vi "Motion_Pulse Coils.vi"(8 "error in":errorcluster, 10 "Pulse Coil":T1=1 items=["GANTRY_ALARM_CLEAR", "GANTRY_ENABLE", "GANTRY_HOME", "GANTRY_GOTO", "LOADER_HOME", "LOADER_ALARM_CLEAR", "LOADER_ENABLE", "LOADER_GOTO_CONNECT", "LOADER_GOTO_LOAD", "LOADER_STOP"], 11 "TCP refnum":refnum<k5>) -> (0 "error out":errorcluster, 3 "TCP refnum dup":refnum<k5>)   [LabVIEW 2010]
uses:
  Motion_Coils Typedef.ctl
  <vilib>/NI Modbus.llb/MB Ethernet Master Query Write Single Coil (poly).vi
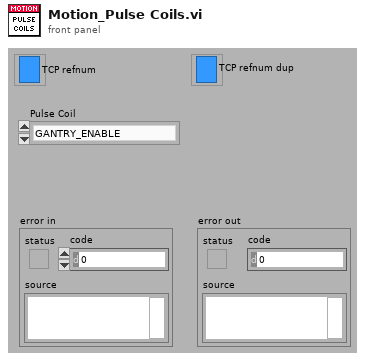
[diagram p1: front panel]
types:
  T1 = typedef "Motion_Coils Typedef.ctl" = u16
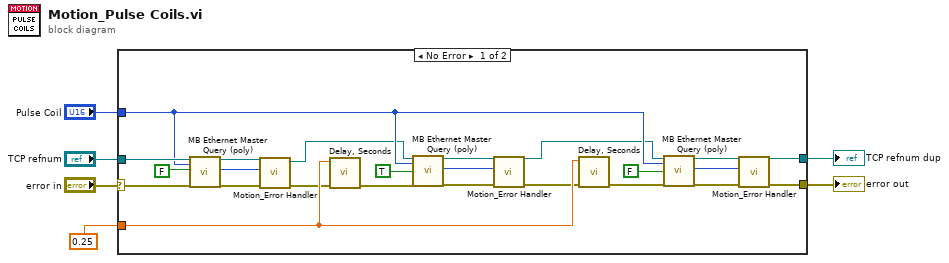
[diagram p0: block diagram]
diagram:
  n1 = case shown="No Error" "error in" {
    selector: "error in" -> [w23 w32]
    tunnel: "Pulse Coil" -> [w22 _]
    tunnel: dbl[unit] 0.25 ("delay") -> [w26 _]
    tunnel: [w13 w32] -> w5
    tunnel: "TCP refnum" -> [w25 w31]
    tunnel: [w11 w31] -> w1
    frame No Error {
      n2 = call-poly <vilib>:"MB Ethernet Master Query (poly).vi"("TCP Connection Refnum in"=w25, "Address"=w22, "Coil"=FALSE, "error in"=w23) -> ("TCP Connection Refnum (dup)"=w21:refnum<k5>, "Exception Code"=w19:u8, "error out"=w18:errorcluster)  [unwired: 13 in]
      n3 = call "Motion_Error Handler.vi"("error in (no error)"=w18, "Exception Code"=w19, "TCP Connection Refnum in"=w21) -> ("error out"=w17:errorcluster, "TCP Connection Refnum (dup)"=w20:refnum<k5>)  [unwired: 7 in]
      n4 = call "Delay, Seconds.vi"("error in"=w17, "delay"=w26) -> ("error out"=w27:errorcluster)  [unwired: 5 in, 1 out]
      n5 = call-poly <vilib>:"MB Ethernet Master Query (poly).vi"("TCP Connection Refnum in"=w20, "Address"=w22, "Coil"=TRUE, "error in"=w27) -> ("TCP Connection Refnum (dup)"=w8:refnum<k5>, "Exception Code"=w9:u8, "error out"=w16:errorcluster)  [unwired: 13 in]
      n6 = call "Motion_Error Handler.vi"("error in (no error)"=w16, "Exception Code"=w9, "TCP Connection Refnum in"=w8) -> ("error out"=w15:errorcluster, "TCP Connection Refnum (dup)"=w7:refnum<k5>)  [unwired: 7 in]
      n7 = call "Delay, Seconds.vi"("error in"=w15, "delay"=w26) -> ("error out"=w29:errorcluster)  [unwired: 5 in, 1 out]
      n8 = call-poly <vilib>:"MB Ethernet Master Query (poly).vi"("TCP Connection Refnum in"=w7, "Address"=w22, "Coil"=FALSE, "error in"=w29) -> ("TCP Connection Refnum (dup)"=w12:refnum<k5>, "Exception Code"=w10:u8, "error out"=w14:errorcluster)  [unwired: 13 in]
      n9 = call "Motion_Error Handler.vi"("error in (no error)"=w14, "Exception Code"=w10, "TCP Connection Refnum in"=w12) -> ("error out"=w13:errorcluster, "TCP Connection Refnum (dup)"=w11:refnum<k5>)  [unwired: 7 in]
    }
    frame Error {
    }
  }
  "error out" <- w5
  "TCP refnum dup" <- w1
